vi "MP_newsetup_Host3.vi"() -> ()   [LabVIEW 2019]
uses:
  <vilib>/rvi/interface/nirviMethod/nirviMethod.xnode
  <vilib>/rvi/errors/niLvFpgaMergeErrorWithErrorCode.vi
  <vilib>/rvi/interface/nirviReadWriteControl/nirviReadWriteControl.xnode
  <vilib>/rvi/interface/Simulation/niFpgaSimulationCallBeginRW.vi
  <vilib>/rvi/errors/niLvFpgaAdjustHostInterfaceError.vi
  <vilib>/Utility/file.llb/Write Delimited Spreadsheet (DBL).vi
  <vilib>/Analysis/NI_AALBase.lvlib
  <vilib>/Analysis/baseanly.llb/Mean (DBL).vi
  <vilib>/FPGAPlugInAG/Dynamic/niLvFpga_Reset_Dynamic.vi
  <vilib>/FPGAPlugInAG/Dynamic/niLvFpga_Run_Dynamic.vi
  <vilib>/rvi/interface/nirviCloseFPGA/nirviCloseFPGA.xnode
  <vilib>/rvi/interface/nirviOpenFPGA/nirviOpenFPGA.xnode
  <vilib>/FPGAPlugInAG/Dynamic/niLvFpga_ConfigureFifo_Dynamic.vi
  <vilib>/FPGAPlugInAG/Dynamic/niLvFpga_StartFifo_Dynamic.vi
  <vilib>/FPGAPlugInAG/Dynamic/niLvFpga_ReadFifo_Dynamic.vi
  <vilib>/FPGAPlugInAG/Dynamic/niLvFpga_StopFifo_Dynamic.vi
  <vilib>/FPGAPlugInAG/Dynamic/niLvFpga_Close_Dynamic.vi
panel:
  in  "cdfnorm":sgl=1.686
  out "num of protocols":sgl
  in  "Collect Xcorr":bool=TRUE
  in  "Calibration ON/OFF":bool=TRUE
  in  "Xoffset":sgl=-0.00173
  in  "Yoffset":sgl=-0.00319
  in  "sum_offset":sgl=-0.0081
  out "Xpot":sgl=-0.6167747 format="%.2f"
  in  "TL":fxp<+/-,20,5>=2.5
  in  "DL":fxp<+/-,20,5>=2.5
  in  "wait time":u8=50
  in  "Temp":i8(ring)=2 items=["Cold", "Warm", "Hot"]
  in  "?":u16(ring)=1 items=["No FB", "FB"]
  in  "Save Xpot":bool=TRUE
  out "PD_TL":dbl(graph)
  out "Xcorr":sgl(graph)
  in  "DW":cluster{"xm":sgl, "Eb":sgl, "Tau":sgl, "dE":sgl}={"xm"=0.5, "Eb"=0.0033, "Tau"=70.0, "dE"=0.0033} {"dE" format="%#_3g"}
  in  "DL_Y":dbl=2.5 format="%#_13g"
  in  "TL_Y":dbl=2.5 format="%#_13g"
  in  "?":bool
  in  "FB time":u32=10
  in  "Triangle wave":T1={"signal offset_X"=5.0, "Scale X"=0.0, "signal offset_Y"=5.0, "Scale Y"=0.0, "Phase Shift"=30}
  in  "Elements":u32=100000
  in  "Data length":dbl=125.0
  out "Done saving":bool
  out "?":dbl=-2.0
  in  "Save Data":bool
  in  "mobX(px/V)":sgl=80.189
  in  "1/Xcali":sgl=-14.3419
  in  "DX":sgl=32.593
  in  "Zstage":fxp<+/-,20,5>=5.29998779296875 format="%#_4g"
  out "Feedback Loop time":sgl=10.0 format="%.2f"
  out "Underflow":bool
  out "X":waveform(dbl)(graph)={"t0"=timestamp(0 s since 1904-01-01), "dt"=9.999999747378752e-06, "Y"=array[100000 elements]}
  out "Y":waveform(dbl)(graph)={"t0"=timestamp(0 s since 1904-01-01), "dt"=9.999999747378752e-06, "Y"=array[100000 elements]}
  out "Sum":waveform(dbl)(graph)={"t0"=timestamp(0 s since 1904-01-01), "dt"=9.999999747378752e-06, "Y"=array[100000 elements]}
  in  "Reaverage PS":bool
  out "meanX":dbl=0.20338191410790663 format="%0.5f"
  in  "Xmean":sgl=-0.40105
  out "PSX":dynamicdata(graph)=[{"t0"=timestamp(0 s since 1904-01-01), "dt"=1.0000000252621255, "Y"=array[50000 elements], "attributes"=variant("NI_ChannelName"=variant(string "PSD"))}]
  out "PSY":dynamicdata(graph)=[{"t0"=timestamp(0 s since 1904-01-01), "dt"=1.0000000252621255, "Y"=array[50000 elements], "attributes"=variant("NI_ChannelName"=variant(string "PSD"))}]
  out "PSsum":dynamicdata(graph)=[{"t0"=timestamp(0 s since 1904-01-01), "dt"=1.0000000252621255, "Y"=array[50000 elements], "attributes"=variant("NI_ChannelName"=variant(string "PSD"))}]
  out "Saveloop":u32
  in  "Feedback parameters":T2={"SP_QPDX"=0.0, "alpha"=0.05, "ktrap"=62.04, "alphacounterX"=0.0218504}
  in  "?":cluster{"SP":sgl, "P":sgl, "I":sgl}={"SP"=0.25, "P"=1.0, "I"=8e-06}
  in  "TW freq":dbl=1.0
  in  "?":cluster{"SP":sgl, "P":sgl, "I":sgl}={"SP"=0.22, "P"=1.0, "I"=5e-06}
  in  "Normalize signal":bool=TRUE
  out "meanY":dbl=0.2228029616717861 format="%0.5f"
  out "meanZ":dbl=0.7304303216481208 format="%0.4f"
  out "?":errorcluster
  in  "file path (dialog if empty)":path=path "C:/Users/Diffusivity/OneDrive - sfu.ca/Mpemba/Data/12-April-2019/t.txt"
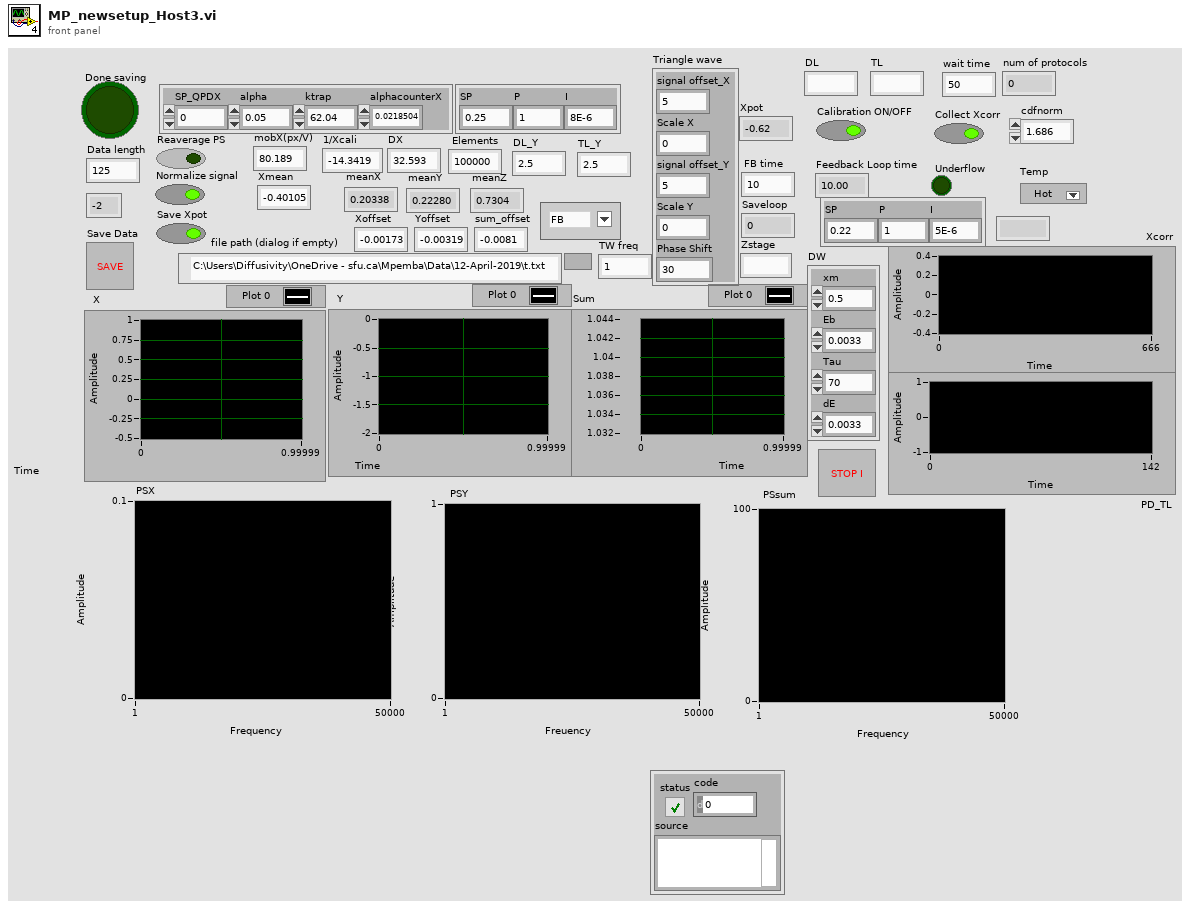
[diagram p1: front panel]
types:
  T1 = cluster{"signal offset_X":sgl, "Scale X":sgl, "signal offset_Y":sgl, "Scale Y":sgl, "Phase Shift":u32}
  T2 = cluster{"SP_QPDX":sgl, "alpha":sgl, "ktrap":sgl, "alphacounterX":sgl}
  T3 = cluster{"signal offset_X":sgl, "Scale X":sgl, "signal offset_Y":sgl, "Scale Y":sgl, u32}
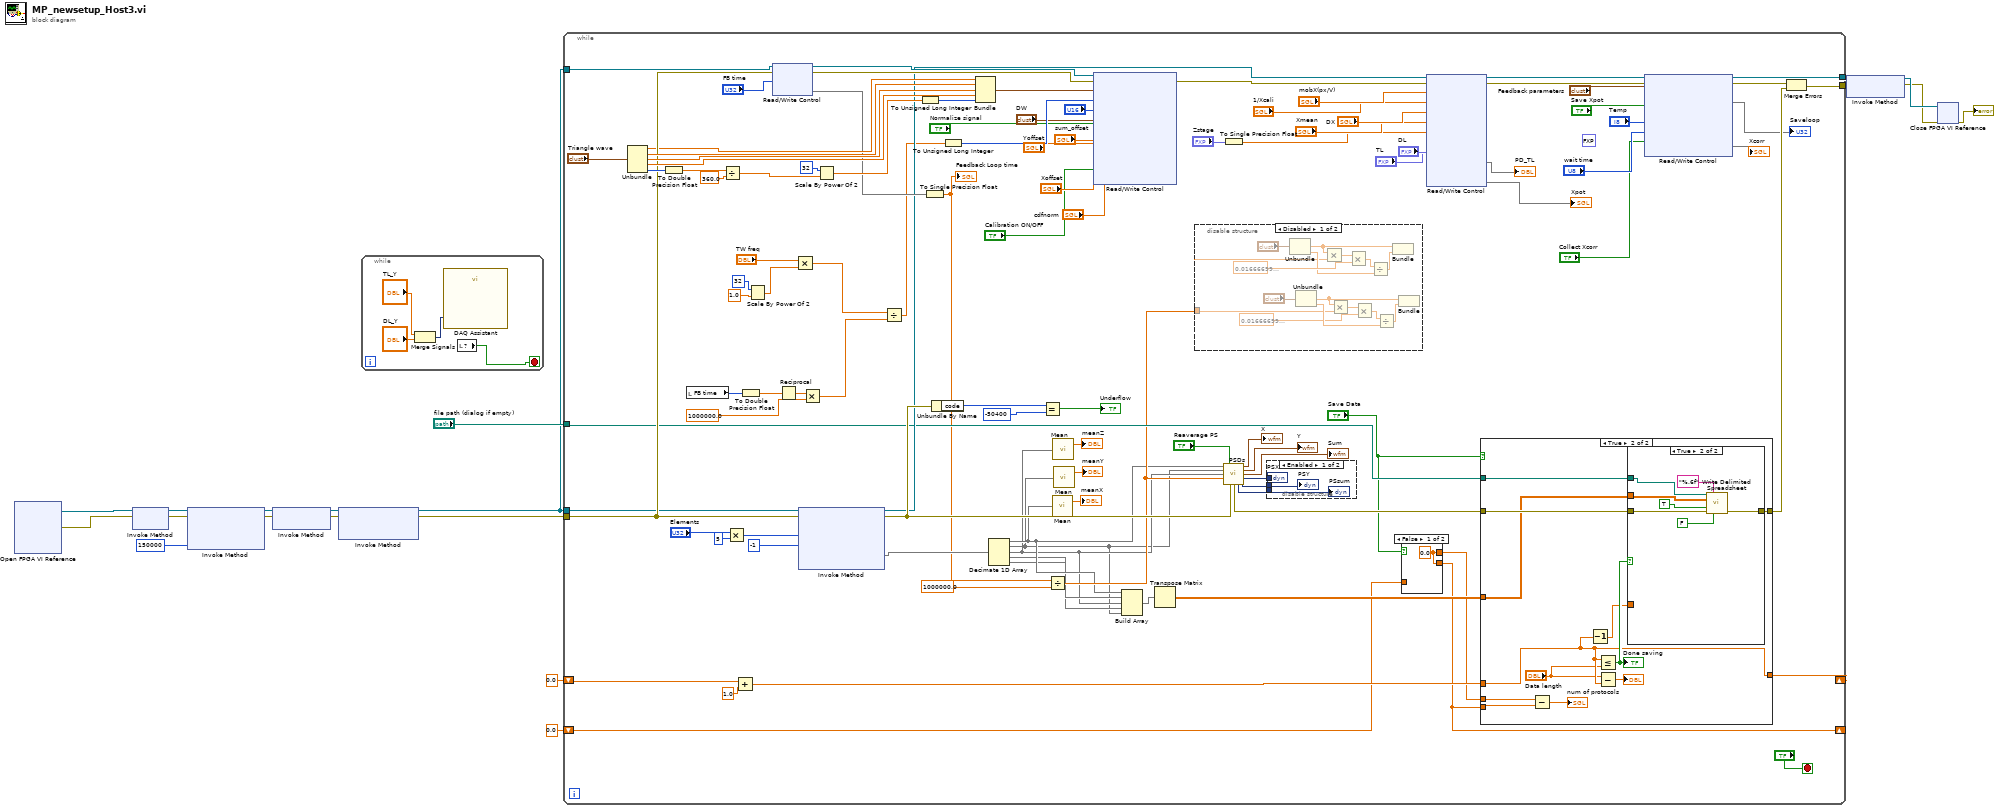
[diagram p0: block diagram]
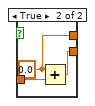
[diagram p3: hidden frame]
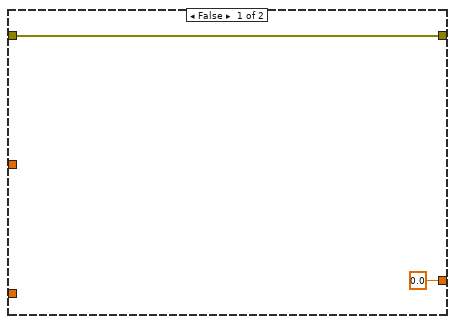
[diagram p5: hidden frame]
diagram:
  n1 = xnode "Open FPGA VI Reference"() -> ("FPGA VI Reference Out"=w2:refnum<k20>, "error out"=w1:errorcluster)  [unwired: 2 in]
  n2 = xnode "Invoke Method"("FPGA VI Reference In"=w2, "error in"=w1) -> ("FPGA VI Reference Out"=w9:refnum<k20>, "error out"=w8:errorcluster)
  n3 = xnode "Invoke Method"("FPGA VI Reference In"=w9, "error in"=w8, "Requested Depth"=u32 150000) -> ("FPGA VI Reference Out"=w14:refnum<k20>, "error out"=w13:errorcluster)  [unwired: 1 out]
  n4 = xnode "Invoke Method"("FPGA VI Reference In"=w14, "error in"=w13) -> ("FPGA VI Reference Out"=w16:refnum<k20>, "error out"=w15:errorcluster)
  n5 = xnode "Invoke Method"("FPGA VI Reference In"=w16, "error in"=w15) -> ("FPGA VI Reference Out"=w12:refnum<k20>, "error out"=w11:errorcluster)  [unwired: 1 in]
  n6 = while {
    stop <- w20 stop-if-true
    n7 = Merge Signals("TL_Y", "DL_Y") -> (w23:dynamicdata)
    n8 = call "DAQ Assistant"("data"=w23) -> ()  [unwired: 17 in, 2 out]
    n9 = local read item#32() -> (w20:bool)
  }
  n10 = while {
    tunnel: w12 -> [w104]
    tunnel: w11 -> [w105]
    tunnel: "file path (dialog if empty)" -> [w69]
    tunnel: [w96] -> w18
    tunnel: [w110] -> w17
    tunnel: w12 -> [w90]
    shift-right: [w101] -> _
    shift-left: 0.0 -> [w100]
    shift-right: [w26] -> _
    shift-left: sgl 0.0 ("num of cycles") -> [w28]
    stop <- "?" stop-if-true
    (unwired) fxp<+,8,7> 50.0 ("Fmax")
    n11 = Unbundle("Triangle wave") -> ("signal offset_X"=w93:sgl, "Scale X"=w114:sgl, "signal offset_Y"=w113:sgl, "Scale Y"=w112:sgl, "Phase Shift"=w115:u32)
    n12 = To Double Precision Float(number=w115) -> (double precision float=w121:dbl)
    n13 = local read "FB time"() -> (w59:u32)
    n14 = Divide(x=w121, y=360.0) -> (x/y=w119:dbl)
    n15 = Multiply(x="Elements", y=u32 5) -> (x*y=w106:u32)
    n16 = Add(x=w100, y=1.0) -> (x+y=w102:dbl)
    n17 = To Double Precision Float(number=w59) -> (double precision float=w60:dbl)
    n18 = Scale By Power Of 2(n=i16 32, x=1.0) -> (x*2^n=w64:dbl)
    n19 = xnode "Read/Write Control"("FPGA VI Reference In"=w104, "error in"=w105, "FB Time"="FB time") -> ("FPGA VI Reference Out"=w126:refnum<k20>, "error out"=w91:errorcluster, "FB Time"=w89)
    n20 = Reciprocal(x=w60) -> (1/x=w61:dbl)
    n21 = Multiply(x="TW freq", y=w64) -> (x*y=w57:dbl)
    n22 = xnode "Invoke Method"("FPGA VI Reference In"=w90, "error in"=w105, "Number of Elements"=w106, "Timeout (ms)"=-1) -> ("FPGA VI Reference Out"=w72:refnum<k20>, "error out"=w87:errorcluster, "Data"=w82:void[])  [unwired: 1 out]
    n23 = Multiply(x=w61, y=1000000.0) -> (x*y=w56:dbl)
    n24 = Scale By Power Of 2(n=i16 32, x=w119) -> (x*2^n=w117:dbl)
    n25 = Divide(x=w57, y=w56) -> (x/y=w55:dbl)
    n26 = To Unsigned Long Integer(number=w117) -> (unsigned 32bit integer=w111:u32)
    n27 = To Single Precision Float(number=w89) -> (single precision float=w66:sgl)
    "Feedback Loop time" <- w66
    n28 = Unbundle By Name(w87) -> ("code"=w109:i32)
    n29 = To Unsigned Long Integer(number=w55) -> (unsigned 32bit integer=w54:u32)
    n30 = Bundle("signal offset_X"=w93, "Scale X"=w114, "signal offset_Y"=w113, "Scale Y"=w112, w111) -> (w67:T3)  [unwired: 1 in]
    n31 = Decimate 1D Array(w82) -> (w48:void[], w35:void[], w46:void[], w36:void[], w47:void[])
    n32 = Equal?(x=w109, y=-50400) -> (x = y?=→"Underflow":bool)
    n33 = Divide(x=w66, y=sgl 1000000.0) -> (x/y=w49:sgl)
    n34 = call-poly <vilib>:"Mean.vi"("X"=w48) -> ("mean"=→"meanX":dbl)  [unwired: 1 out]
    n35 = call-poly <vilib>:"Mean.vi"("X"=w46) -> ("mean"=→"meanZ":dbl)  [unwired: 1 out]
    n36 = call-poly <vilib>:"Mean.vi"("X"=w35) -> ("mean"=→"meanY":dbl)  [unwired: 1 out]
    n37 = xnode "Read/Write Control"("FPGA VI Reference In"=w126, "error in"=w91, "Triangle wave"=w67, "Frequency"=w54, "Enum"="?", "DW"="DW", "Normalize signal"="Normalize signal", "sum_offset"="sum_offset", "Yoffset"="Yoffset", "Xoffset"="Xoffset", "Calibration ON/OFF"="Calibration ON/OFF", "cdfnorm"="cdfnorm") -> ("error out"=w71:errorcluster)  [unwired: 1 out]
    n38 = Build Array(w48, w47, w46, w36, w35) -> (w94:void[])
    n39 = Transpose Matrix(1:w94) -> (0:w124:dbl[][])
    n40 = disable-structure shown="Disabled" {
      disable-tunnel: w49 -> [w130 _]
      frame Disabled {
        n41 = Unbundle("?") -> ("P"=w138:sgl, "I"=w139:sgl)  [unwired: 1 out]
        n42 = Unbundle("?") -> ("P"=w135:sgl, "I"=w134:sgl)  [unwired: 1 out]
        n43 = Multiply(x=w138, y=w130) -> (x*y=w142:sgl)
        n44 = Multiply(x=w135, y=w130) -> (x*y=w132:sgl)
        n45 = Multiply(x=w142, y=sgl 0.016667) -> (x*y=w140:sgl)
        n46 = Multiply(x=w132, y=sgl 0.016667) -> (x*y=w133:sgl)
        n47 = Divide(x=w140, y=w139) -> (x/y=w137:sgl)
        n48 = Divide(x=w133, y=w134) -> (x/y=w136:sgl)
        n49 = Bundle("P"=w138, w137) -> ()  [unwired: 1 in, 1 out]
        n50 = Bundle("P"=w135, w136) -> ()  [unwired: 1 in, 1 out]
      }
      frame Enabled {
      }
    }
    n51 = call "PSDs.vi"("X"=w48, "averaging done"="Reaverage PS", "Y"=w35, "sum"=w46, "dt"=w49, "error in (no error)"=w87) -> ("X"=→"X":waveform(dbl), "Y"=→"Y":waveform(dbl), "Sum"=→"Sum":waveform(dbl), "PSDX"=w78:dynamicdata, "error out"=w86:errorcluster, "PSDsum"=w76:dynamicdata, "PSDY"=w77:dynamicdata)  [unwired: 3 in]
    n52 = To Single Precision Float(number="Zstage") -> (single precision float=w70:sgl)
    n53 = disable-structure shown="Enabled" {
      disable-tunnel: w78 -> [w150 _]
      disable-tunnel: w77 -> [w149 _]
      disable-tunnel: w76 -> [w148 _]
      frame Enabled {
        "PSX" <- w150
        "PSY" <- w149
        "PSsum" <- w148
      }
      frame Disabled {
      }
    }
    n54 = case shown="False" "Save Data" {
      tunnel: [w144 w146] -> w26
      tunnel: w28 -> [_ w147]
      tunnel: [w144 w145] -> w27
      frame False {
        w144 = sgl 0.0 ("num of cycles")
      }
      frame True {
        w145 = sgl 0.0 ("num of cycles")
        n55 = Add(x=w145, y=w147) -> (x+y=w146:sgl)
      }
    }
    n56 = xnode "Read/Write Control"("FPGA VI Reference In"=w72, "error in"=w71, "MobX(px/V)"="mobX(px/V)", "1/Xcali"="1/Xcali", "DX"="DX", "Xmean"="Xmean", "Zstage_offset"=w70, "DL"="DL", "TL"="TL") -> ("FPGA VI Reference Out"=w98:refnum<k20>, "error out"=w97:errorcluster, "PD_T"=→"PD_TL", "Xpot"=→"Xpot")  [unwired: 1 out]
    n57 = case shown="True" "Save Data" {
      tunnel: w124 -> [_ w159]
      tunnel: w69 -> [_ w164]
      tunnel: w86 -> [w152 w163]
      tunnel: [w152 w162] -> w123
      tunnel: w102 -> [_ w158]
      tunnel: [0.0 w158] -> w101
      tunnel: w27 -> [_ w155]
      tunnel: w26 -> [_ w154]
      frame False {
      }
      frame True {
        n58 = Subtract(x=w155, y=w154) -> (x-y=→"num of protocols":sgl)
        n59 = Decrement(x=w158) -> (x-1=w157:dbl)
        n60 = Less Or Equal?(x=w158, y="Data length") -> (x <= y?=w161:bool)
        "Done saving" <- w161
        n61 = Subtract(x="Data length", y=w158) -> (x-y=→"?":dbl)
        n62 = case shown="True" w161 {
          tunnel: w159 -> [_ w166]
          tunnel: w164 -> [_ w167]
          tunnel: w163 -> [w165 w170]
          tunnel: [w165 w169] -> w162
          tunnel: w157 -> [_ _]
          frame False {
          }
          frame True {
            n63 = call-poly <vilib>:"Write Delimited Spreadsheet.vi"("file path (dialog if empty)"=w167, "format (%.3f)"="%.6f", "2D data"=w166, "append to file? (new file:F)"=TRUE, "error in (no error)"=w170, "transpose? (no:F)"=FALSE) -> ("error out"=w169:errorcluster)  [unwired: 8 in, 1 out]
          }
        }
      }
    }
    n64 = xnode "Read/Write Control"("FPGA VI Reference In"=w98, "error in"=w97, "Feedback parameters"="Feedback parameters", "Save Xpot"="Save Xpot", "Temp"="Temp", "wait time"="wait time", "Collect Xcorr"="Collect Xcorr") -> ("FPGA VI Reference Out"=w96:refnum<k20>, "error out"=w95:errorcluster, "Saveloop"=→"Saveloop", "xcorr"=→"Xcorr")
    n65 = Merge Errors(w95, w123) -> (w110:errorcluster)
  }
  n66 = xnode "Invoke Method"("FPGA VI Reference In"=w18, "error in"=w17) -> ("FPGA VI Reference Out"=w7:refnum<k20>, "error out"=w6:errorcluster)
  n67 = xnode "Close FPGA VI Reference"("FPGA VI Reference In"=w7, "error in"=w6) -> ("error out"=→"?":errorcluster)
